vi "Actor Core.vi"(8 "error in (no error)":errorcluster, 11 "Mag Lab Measure Interface in":refnum<class "XY Plot.lvclass">) -> (0 "error out":errorcluster, 3 "Actor Framework.lvlib:Actor":refnum<class "Actor.lvclass">)   [LabVIEW 2015, in "XY Plot.lvclass"]
uses:
  XY Plot.lvclass
  <vilib>/ActorFramework/Stop Msg/Stop Msg.lvclass
  <vilib>/ActorFramework/Actor/Actor.lvclass
  XY Plot Messages/Add file Msg/Add file Msg.lvclass
  XY Plot Messages/Replot Msg/Replot Msg.lvclass
  XY Plot Messages/Save keep old plots Msg/Save keep old plots Msg.lvclass
  XY Plot Messages/Save defaults Msg/Save defaults Msg.lvclass
  Plot/Plot.lvclass
panel:
  in  "Set as default":bool
  in  "Keep old\nplots":bool
  in  "Open":bool
  in  "Exit":bool
  in  "Plots":cluster{"X":u16, "Y":u16}[](array[cluster]) {"Y" items=["Select channel...", "Time", "Y"]; "X" items=["Select channel...", "Time", "Y"]}
  out "XY Graph":cluster{dbl[], dbl[]}[](graph)
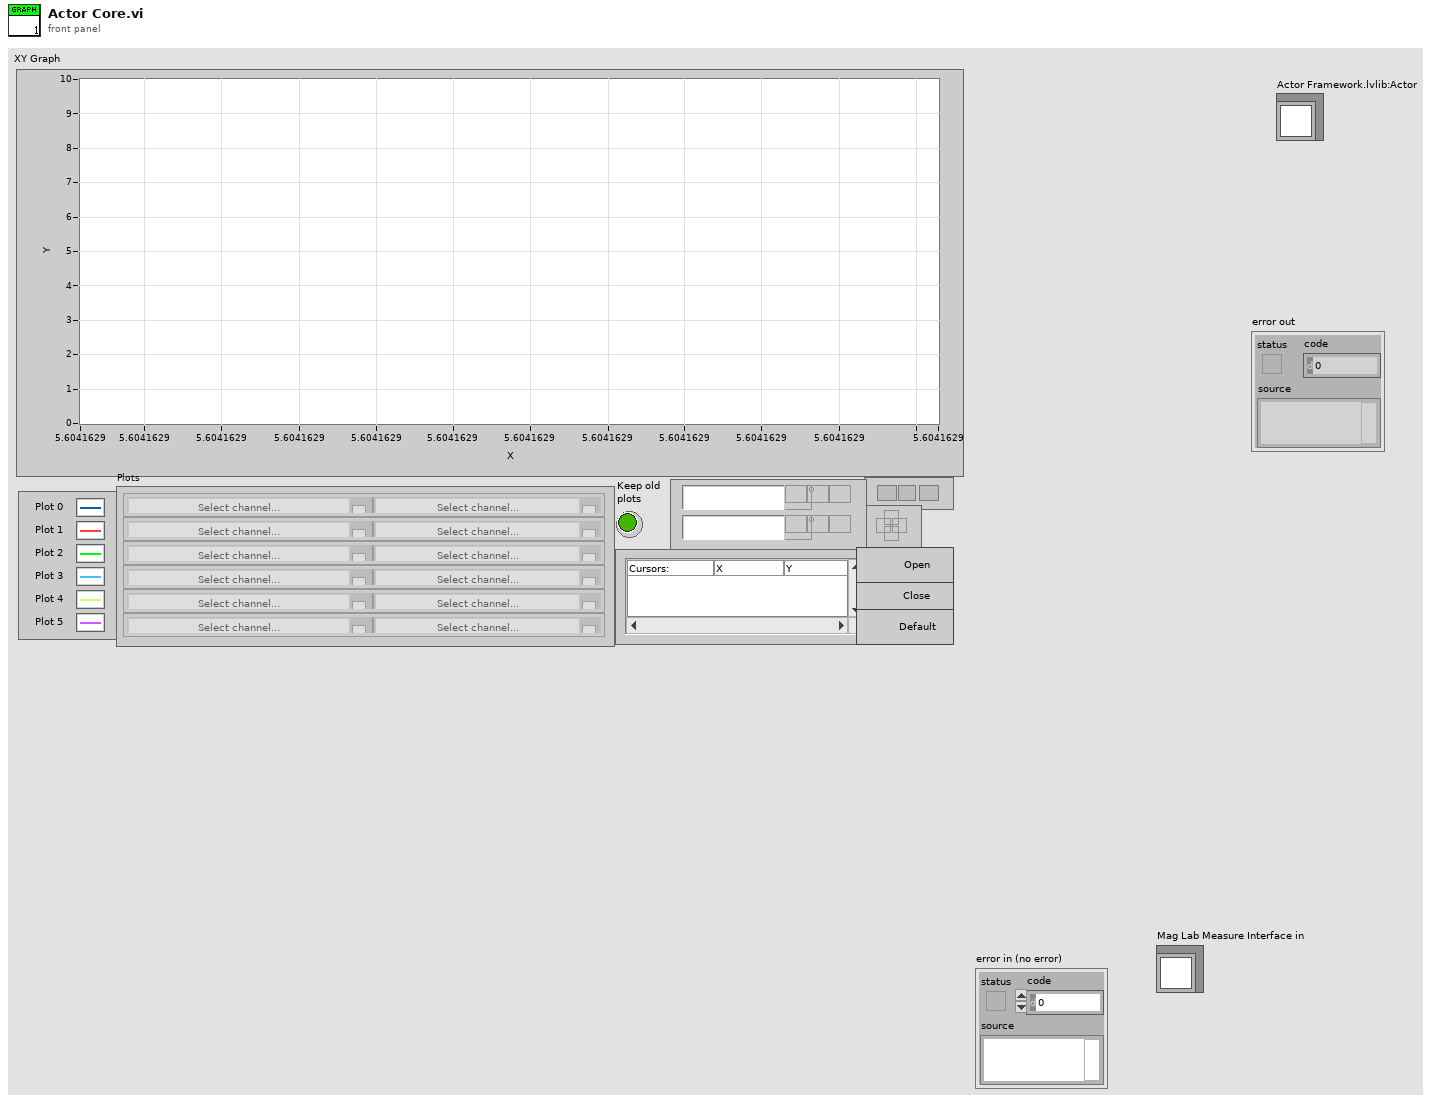
[diagram p1: front panel]
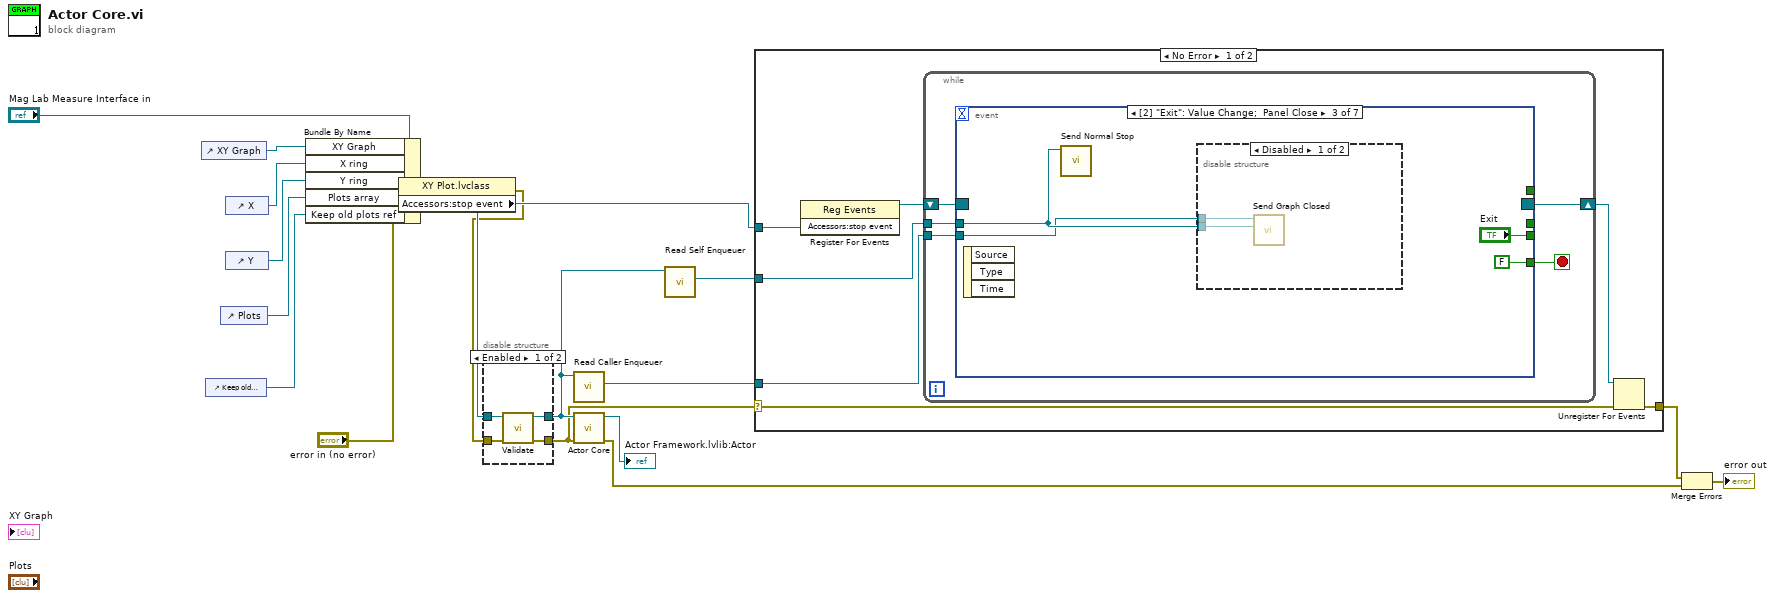
[diagram p0: block diagram]
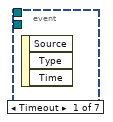
[diagram p3: hidden frame]
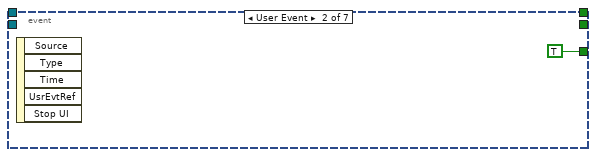
[diagram p4: hidden frame]
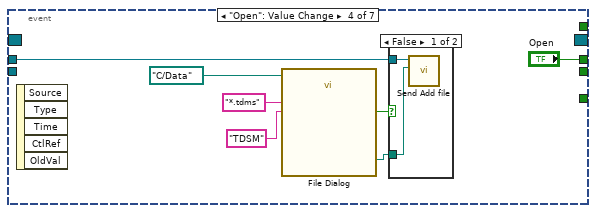
[diagram p6: hidden frame]
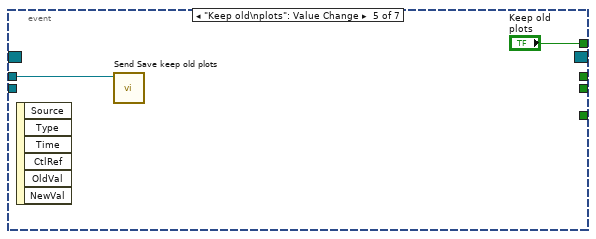
[diagram p8: hidden frame]
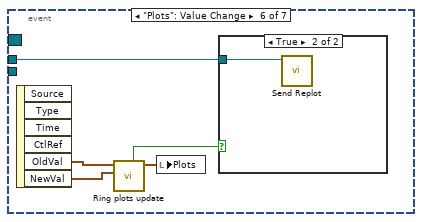
[diagram p9: hidden frame]
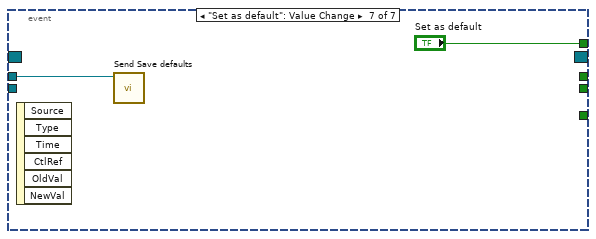
[diagram p11: hidden frame]
diagram:
  n1 = control-ref of="XY Graph"() -> (w12:refnum<vi>)
  n2 = control-ref of="Keep old\nplots"() -> (w9:refnum<vi>)
  n3 = control-ref of="Plots"() -> (w15:refnum<vi>)
  n4 = control-ref of="X"() -> (w14:refnum<vi>)
  n5 = control-ref of="Y"() -> (w13:refnum<vi>)
  n6 = Bundle By Name(cluster="Mag Lab Measure Interface in", "XY Graph"=w12, "X ring"=w14, "Y ring"=w13, "Plots array"=w15, "Keep old plots ref"=w9) -> (w5:refnum<class "XY Plot.lvclass">)
  n7 = property class="XY Plot.lvclass"(reference=w5, error in="error in (no error)") -> (reference out=w4:refnum<class "XY Plot.lvclass">, error out=w1:errorcluster, "Accessors:stop event"=w3:refnum<user-event>)
  n8 = disable-structure shown="Enabled" {
    disable-tunnel: [w23 w25] -> w8
    disable-tunnel: [w22 w24] -> w10
    disable-tunnel: w1 -> [w21 w25]
    disable-tunnel: w4 -> [w20 w24]
    frame Enabled {
      n9 = call-dynamic "Validate.vi"("error in (no error)"=w21, "MagLabGraph in"=w20) -> ("error out"=w23:errorcluster, "MagLabGraph out"=w22:refnum<class "XY Plot.lvclass">)  [unwired: 8 in]
    }
    frame Disabled {
    }
  }
  n10 = call <vilib>:"Read Caller Enqueuer.vi"("Actor"=w10) -> ("Caller Enqueuer"=w11:refnum<class "Message Enqueuer.lvclass">)  [unwired: 10 in]
  n11 = call-parent "Actor Core.vi"("error in"=w8, "Measure Object in"=w10) -> ("error out"=w6:errorcluster, "Actor out"=→"Actor Framework.lvlib:Actor":refnum<class "Actor.lvclass">)  [unwired: 8 in]
  n12 = call <vilib>:"Read Self Enqueuer.vi"("Actor"=w10) -> ("Self Enqueuer"=w17:refnum<class "Message Enqueuer.lvclass">)  [unwired: 10 in]
  n13 = case shown="No Error" w8 {
    selector: w8 -> [w26 w64]
    tunnel: w3 -> [w31 _]
    tunnel: w17 -> [w30 _]
    tunnel: [w29 w64] -> w16
    tunnel: w11 -> [w27 _]
    frame No Error {
      n14 = register-events(w31) -> (reference out=w32:refnum<event-registration>)  [unwired: 2 in, 1 out]
      n15 = while {
        tunnel: w30 -> [w36]
        shift-right: [w34] -> w28
        shift-left: w32 -> [w37]
        tunnel: w27 -> [w33]
        stop <- w35 stop-if-true
        n16 = event shown="[2] \"Exit\": Value Change;  Panel Close" {
          selector: w37 -> [_ _ _ _ _ _ _]
          dyn-events: [_ _ _ _ _ _ _] -> w34
          timeout: _ -> [_ _ _ _ _ _ _]
          tunnel: w36 -> [_ _ w40 w46 w55 w56 w62]
          tunnel: [_ TRUE FALSE _ _ _ _] -> w35
          tunnel: [_ _ "Exit" _ _ _ _] -> _
          tunnel: [_ _ _ "Open" _ _ _] -> _
          tunnel: w33 -> [_ _ w39 _ _ _ _]
          tunnel: [_ _ _ _ "Keep old\nplots" _ "Set as default"] -> _
          event Timeout {
            n17 = event-data() -> ()  [unwired: 1 in, 3 out]
          }
          event User Event {
            n18 = event-data() -> ()  [unwired: 1 in, 5 out]
          }
          event "Exit": Value Change; Panel Close {
            n19 = event-data() -> ()  [unwired: 1 in, 3 out]
            n20 = call <vilib>:"Send Normal Stop.vi"("Message Enqueuer"=w40) -> ()  [unwired: 10 in, 1 out]
            n21 = disable-structure shown="Disabled" {
              disable-tunnel: w40 -> [w44 _]
              disable-tunnel: w39 -> [w43 _]
              frame Disabled {
                n22 = call "Send Graph Closed.vi"("Closed Graph"=w44, "Message Enqueuer"=w43) -> ()  [unwired: 8 in, 2 out]
              }
              frame Enabled {
              }
            }
          }
          event "Open": Value Change {
            n23 = event-data() -> ()  [unwired: 1 in, 5 out]
            n24 = call "File Dialog"("start path"=path "C:/Data", "pattern (all files)"="*.tdms", "pattern label"="TDSM") -> ("selected path"=w45:path, "cancelled"=w47:bool)  [unwired: 9 in, 2 out]
            n25 = case shown="False" w47 {
              tunnel: w46 -> [w53 _]
              tunnel: w45 -> [w52 _]
              frame False {
                n26 = call "Send Add file.vi"("File Path Control"=w52, "Message Enqueuer"=w53) -> ()  [unwired: 8 in, 2 out]
              }
              frame True {
              }
            }
          }
          event "Keep old\nplots": Value Change {
            n27 = event-data() -> ()  [unwired: 1 in, 6 out]
            n28 = call "Send Save keep old plots.vi"("Message Enqueuer"=w55) -> ()  [unwired: 9 in, 2 out]
          }
          event "Plots": Value Change {
            n29 = event-data() -> ("OldVal"=w58:cluster{"X":u16, "Y":u16}[], "NewVal"=w59:cluster{"X":u16, "Y":u16}[])  [unwired: 1 in, 4 out]
            n30 = call "Ring plots update.vi"("New Plots"=w59, "Old Plots"=w58) -> ("Plots"=w60:cluster{"X":u16, "Y":u16}[], "Replot?"=w57:bool)  [unwired: 8 in]
            n31 = local write "Plots"(w60) -> ()
            n32 = case shown="True" w57 {
              tunnel: w56 -> [_ w61]
              frame False {
              }
              frame True {
                n33 = call "Send Replot.vi"("Message Enqueuer"=w61) -> ()  [unwired: 9 in, 2 out]
              }
            }
          }
          event "Set as default": Value Change {
            n34 = event-data() -> ()  [unwired: 1 in, 6 out]
            n35 = call "Send Save defaults.vi"("Message Enqueuer"=w62) -> ()  [unwired: 9 in, 2 out]
          }
        }
      }
      n36 = Unregister For Events(event registration refnum=w28, error in=w26) -> (error out=w29:errorcluster)
    }
    frame Error {
    }
  }
  n37 = Merge Errors(w16, w6) -> (→"error out":errorcluster)
